vi "Ramp Pattern w_1.vi"(2 "start":dbl format="%0.2f", 3 "end":dbl=1.0 format="%0.2f", 4 "samples":i32=128) -> (0 "error":i32, 1 "Ramp Pattern":dbl[](array[numeric]) format="%0.2f")   [LabVIEW 2014]
uses:
  <vilib>/Analysis/1siggen.llb/Ramp Pattern by Samples.vi
  <vilib>/Analysis/NI_AALBase.lvlib
panel:
  # "Ramp Pattern 2"
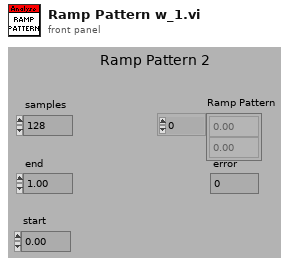
[diagram p1: front panel]
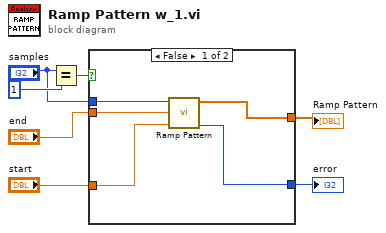
[diagram p0: block diagram]
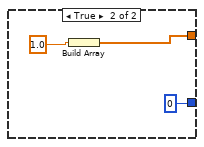
[diagram p2: hidden frame]
diagram:
  n1 = Equal?(x="samples", y=1) -> (x = y?=w6:bool)
  n2 = case shown="False" w6 {
    tunnel: [w8 w14] -> w5
    tunnel: "samples" -> [w12 _]
    tunnel: "end" -> [w11 _]
    tunnel: "start" -> [w10 _]
    tunnel: [w9 0 ("error")] -> w1
    frame False {
      n3 = call-poly <vilib>:"Ramp Pattern.vi"("start"=w10, "end"=w11, "samples"=w12) -> ("error"=w9:i32, "Ramp Pattern"=w8:dbl[])  [unwired: 7 in]
    }
    frame True {
      n4 = Build Array(1.0 ("y")) -> (w14:dbl[])
    }
  }
  "Ramp Pattern" <- w5
  "error" <- w1
